vi "Main.vi"(11 "Module Admin":refnum<class "Delacor_lib_QMH_Module Admin.lvclass">) -> ()   [LabVIEW 2020, in "User Interface.lvlib"]
doc: "This template is based off of the Queued Message Handler design pattern and the Queued Message Handler project template that ships with LabVIEW.\n\nThe main difference is that the queue is private to this module and communication between modules is performed via Broadcast and Request events.\n\nRequest events are wrapped in public API methods and are handled in the Event Handling Loop (EHL) of this VI. Any module can register for Broadcast events sent by this module. The EHL generates messages based on user interface actions.\n\nThe Message Handling Loop (MHL) processes messages generated by the EHL, or by other messages. The messages are string values, so new messages can be added easily to the Message Cases case structure in the MHL. Each message cluster can also provide an optional value for Message Data, which is a variant that can be converted to whatever message-specific data is required.\n_____\nBased on Delacor QMH Project Template 6.0.0.89."
uses:
  User Interface.lvlib
  <vilib>/Delacor/Delacor QMH/Libraries/Module Admin_class/Delacor_lib_QMH_Module Admin.lvclass
  Module Data--cluster.ctl
  Stop Argument--cluster.ctl
  <vilib>/Delacor/Delacor QMH/Libraries/Message Queue_class/Delacor_lib_QMH_Message Queue.lvclass/Delacor_lib_QMH_Message Queue.ctl
  <vilib>/Delacor/Delacor QMH/Libraries/Module Admin_class/Delacor_lib_QMH_Module Admin.lvclass/Delacor_lib_QMH_Module Admin.ctl
  Start Acquisition Argument--cluster.ctl
  Settings Argument--cluster.ctl
  <vilib>/Delacor/Delacor QMH/Libraries/Message Queue_class/Delacor_lib_QMH_Enqueue Message (Single).vi
  <vilib>/Delacor/Delacor QMH/Libraries/Module Admin_class/Delacor_lib_QMH_Get External Launch.vi
  <vilib>/Utility/error.llb/Error Cluster From Error Code.vi
  <vilib>/ErrorRing/Error Ring.xnode
  <vilib>/Delacor/Delacor QMH/Libraries/Message Queue_class/Delacor_lib_QMH_Message Queue.lvclass
  Settings/Settings.lvlib
  Acquisition/Acquisition .lvlib
  Logging/Logging.lvlib
panel:
  out "Analog Signals":waveform(dbl)[](graph)
  out "Status":string
  out "Digital Signals":bool[](array[boolean])
  out "error out":errorcluster
  in  "Stop secuence":bool
  in  "Settings":bool
  in  "Start Secuence":bool
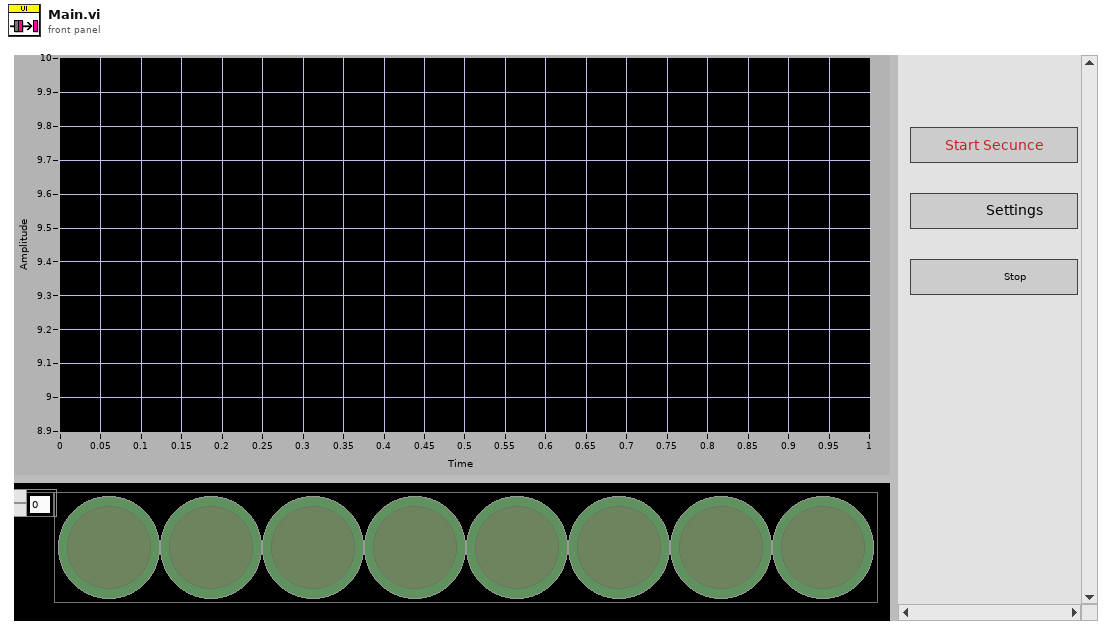
[diagram p1: front panel]
types:
  T1 = typedef "User Interface.lvlib/Request Events--cluster.ctl" = cluster{"Stop Module":refnum<user-event>, "Show Panel":refnum<user-event>, "Hide Panel":refnum<user-event>, "Get Module Execution Status":refnum<user-event>, "Show Diagram":refnum<user-event>, "Start Acquisition":refnum<user-event>, "Settings":refnum<user-event>}
  T2 = typedef "Settings.lvlib/Broadcast Events--cluster.ctl" = cluster{"Module Did Init":refnum<user-event>, "Status Updated":refnum<user-event>, "Error Reported":refnum<user-event>, "Module Did Stop":refnum<user-event>, "Update Module Execution Status":refnum<user-event>, "Config has been set":refnum<user-event>, "Prueba has been set":refnum<user-event>, "Digital has been set":refnum<user-event>}
  T3 = typedef "Acquisition .lvlib/Broadcast Events--cluster.ctl" = cluster{"Module Did Init":refnum<user-event>, "Status Updated":refnum<user-event>, "Error Reported":refnum<user-event>, "Module Did Stop":refnum<user-event>, "Update Module Execution Status":refnum<user-event>, "analog data":refnum<user-event>, "digital data":refnum<user-event>, "Digital Metdata has been acquired":refnum<user-event>}
  T4 = typedef "User Interface.lvlib/Module Data--cluster.ctl" = cluster{"Status":string}
  T5 = enum32{"invalid lock state", "Not Locked", "Locked (No Password)", "Password-protected"}
  T6 = typedef "User Interface.lvlib/Stop Argument--cluster.ctl" = cluster{"Origin":string, "Exit via Stop Module Req?":bool, "Wait for Module to stop?":bool}
  T7 = typedef "User Interface.lvlib/Start Acquisition Argument--cluster.ctl" = cluster{"Start Secuence":bool}
  T8 = typedef "User Interface.lvlib/Settings Argument--cluster.ctl" = cluster{"Settings":bool}
  T9 = enum32{"Invalid", "Standard", "Closed", "Hidden", "Minimized", "Maximized"}
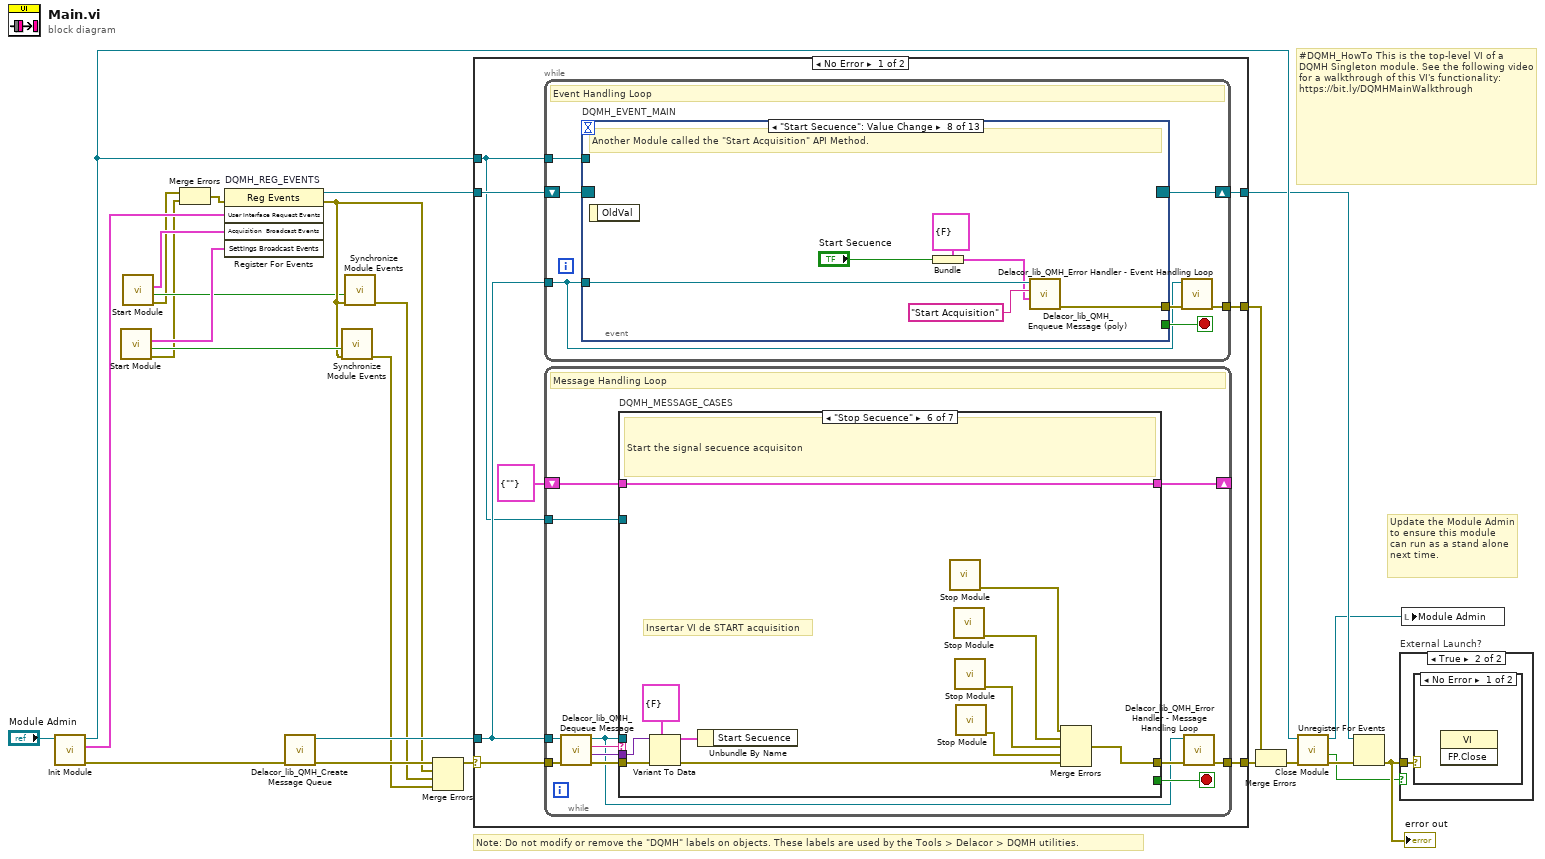
[diagram p0: block diagram]
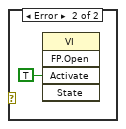
[diagram p3: hidden frame]
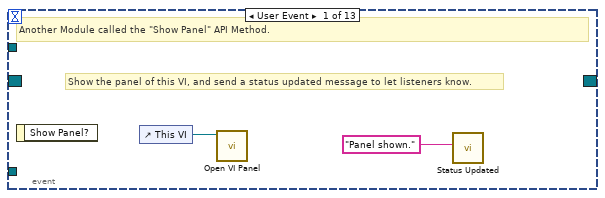
[diagram p4: hidden frame]
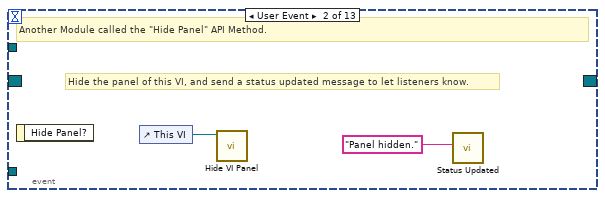
[diagram p5: hidden frame]
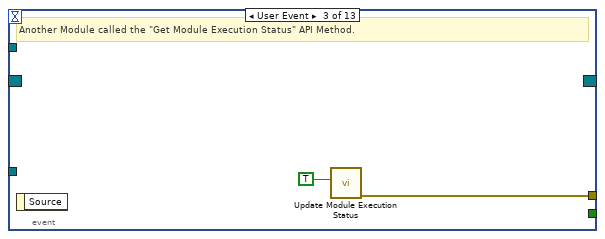
[diagram p6: hidden frame]
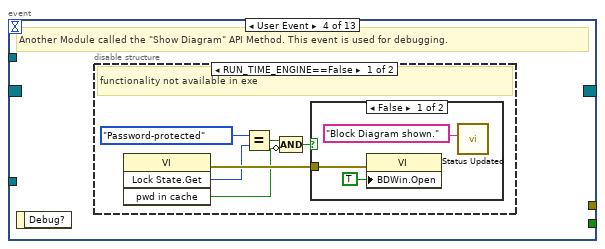
[diagram p7: hidden frame]
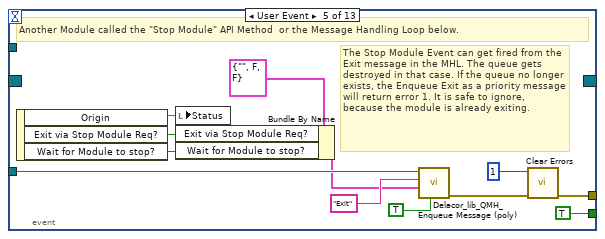
[diagram p10: hidden frame]
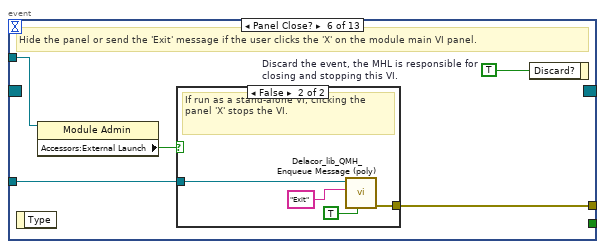
[diagram p11: hidden frame]
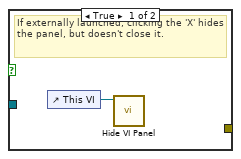
[diagram p12: hidden frame]
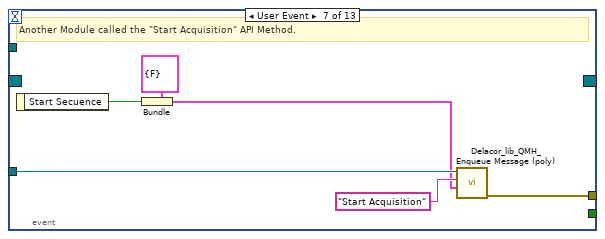
[diagram p13: hidden frame]
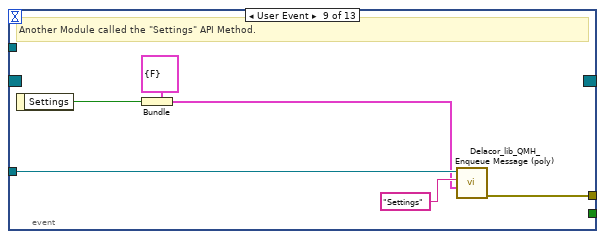
[diagram p14: hidden frame]
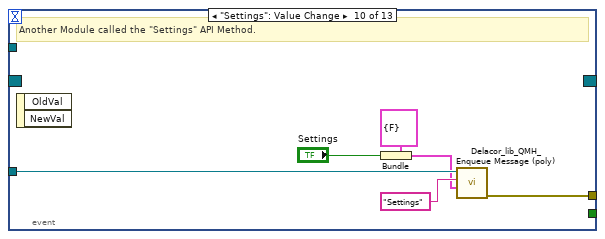
[diagram p15: hidden frame]
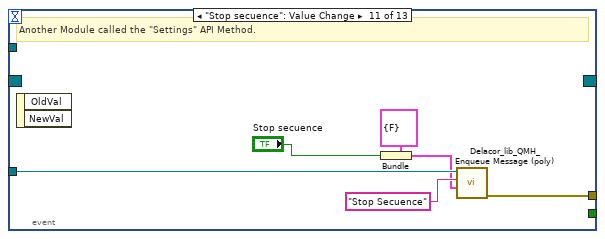
[diagram p16: hidden frame]
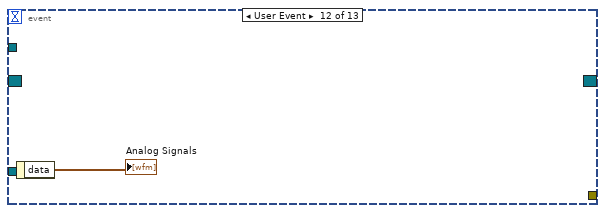
[diagram p17: hidden frame]
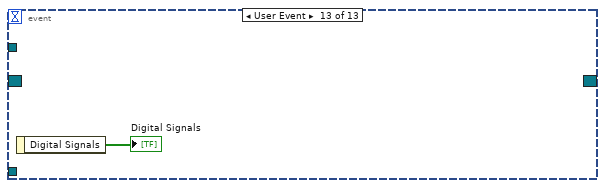
[diagram p18: hidden frame]
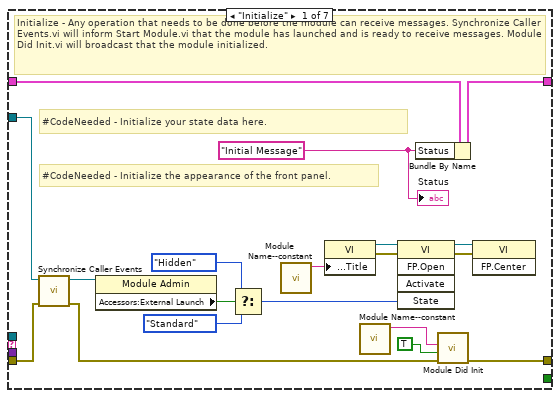
[diagram p19: hidden frame]
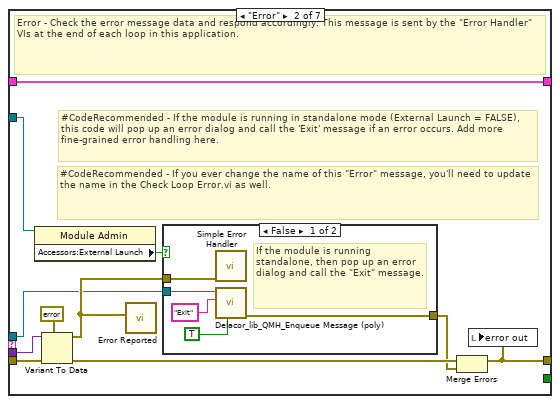
[diagram p20: hidden frame]
diagram:
  # "#DQMH_HowTo This is the top-level VI of a DQMH Singleton module. See the following video for a walkthrough of this VI's functionality: https://bit.ly/DQMHMainWalkthrough"
  # "Note: Do not modify or remove the \"DQMH\" labels on objects. These labels are used by the Tools > Delacor > DQMH utilities."
  # "Update the Module Admin to ensure this module can run as a stand alone next time."
  n1 = call "Init Module.vi"("Singleton Module Admin in"="Module Admin") -> ("error out"=w25:errorcluster, "User Interface Request Events"=w15:T1, "Singleton Module Admin out"=w18:refnum<class "Delacor_lib_QMH_Module Admin.lvclass">)  [unwired: 8 in]
  n2 = call "Start Module.vi"() -> ("error out"=w3:errorcluster, "Wait for Event Sync?"=w10:bool, "Settings Broadcast Events"=w9:T2)  [unwired: 8 in, 1 out]
  n3 = call "Start Module.vi"() -> ("error out"=w5:errorcluster, "Wait for Event Sync?"=w7:bool, "Acquisition  Broadcast Events"=w6:T3)  [unwired: 8 in, 1 out]
  n4 = Merge Errors(w5, w3) -> (w4:errorcluster)
  n5 = register-events "DQMH_REG_EVENTS"(error in=w4, w15, w6, w9) -> (reference out=w16:refnum<event-registration>, error out=w8:errorcluster)  [unwired: 1 in]
  n6 = call <vilib>:"Delacor_lib_QMH_Create Message Queue.vi"("error in"=w25) -> ("error out"=w20:errorcluster, "Message Queue"=w14:refnum<class "Delacor_lib_QMH_Message Queue.lvclass">)  [unwired: 9 in]
  n7 = call "Synchronize Module Events.vi"("error in"=w8, "Wait for Event Sync?"=w10) -> ("error out"=w2:errorcluster)  [unwired: 9 in]
  n8 = call "Synchronize Module Events.vi"("error in"=w8, "Wait for Event Sync?"=w7) -> ("error out"=w1:errorcluster)  [unwired: 9 in]
  n9 = Merge Errors(w20, w8, w1, w2) -> (w19:errorcluster)
  n10 = case shown="No Error" w19 {
    selector: w19 -> [w32 w216]
    tunnel: [w34 w215] -> w26
    tunnel: [w31 w221] -> w17
    tunnel: w16 -> [w29 w221]
    tunnel: w14 -> [w28 w214]
    tunnel: [w33 _] -> w23
    tunnel: w18 -> [w27 w217]
    frame No Error {
      n11 = while {
        tunnel: w28 -> [w35]
        shift-right: [w38] -> w31
        shift-left: w29 -> [w39]
        tunnel: [w40] -> w33
        tunnel: w27 -> [w36]
        stop <- w37 stop-if-true
        # "Event Handling Loop"
        n12 = event "DQMH_EVENT_MAIN" shown="[7] \"Start Secuence\": Value Change" {
          selector: w39 -> [_ _ _ _ _ _ _ _ _ _ _ _ _]
          dyn-events: [_ _ _ _ _ _ _ _ _ _ _ _ _] -> w38
          timeout: _ -> [_ _ _ _ _ _ _ _ _ _ _ _ _]
          tunnel: [_ _ _ _ TRUE ("Discard?") _ _ _ _ _ _ _ _] -> w37
          tunnel: w35 -> [_ _ _ _ w64 w71 w84 w90 w96 w102 w108 _ _]
          tunnel: [_ _ w47 _ w67 w73 w79 w86 w91 w98 w104 _ _] -> w41
          tunnel: w36 -> [_ _ _ _ _ w70 _ _ _ _ _ _ _]
          event User Event {
            # "Show the panel of this VI, and send a status updated message to let listeners know."
            # "Another Module called the \"Show Panel\" API Method."
            n13 = event-data() -> ()  [unwired: 1 in, 1 out]
            n14 = control-ref of="This VI"() -> (w43:refnum<vi>)
            n15 = call "Open VI Panel.vi"("VI"=w43) -> ()  [unwired: 10 in, 1 out]
            n16 = call "Status Updated.vi"("Status"="Panel shown." ("format string")) -> ()  [unwired: 10 in, 1 out]
          }
          event User Event {
            # "Hide the panel of this VI, and send a status updated message to let listeners know."
            # "Another Module called the \"Hide Panel\" API Method."
            n17 = event-data() -> ()  [unwired: 1 in, 1 out]
            n18 = control-ref of="This VI"() -> (w45:refnum<vi>)
            n19 = call "Hide VI Panel.vi"("VI"=w45) -> ()  [unwired: 10 in, 1 out]
            n20 = call "Status Updated.vi"("Status"="Panel hidden." ("format string")) -> ()  [unwired: 10 in, 1 out]
          }
          event User Event {
            # "Another Module called the \"Get Module Execution Status\" API Method."
            n21 = event-data() -> ()  [unwired: 1 in, 1 out]
            n22 = call "Update Module Execution Status.vi"("Running?"=TRUE) -> ("error out"=w47:errorcluster)  [unwired: 10 in]
          }
          event User Event {
            # "Another Module called the \"Show Diagram\" API Method. This event is used for debugging."
            n23 = event-data() -> ()  [unwired: 1 in, 1 out]
            n24 = disable-structure shown="RUN_TIME_ENGINE==False" {
              frame condition #0 (active) {
                # "functionality not available in exe"
                n25 = invoke class="VI" method="Lock State.Get"() -> (error out=w53:errorcluster, "Get Lock State"=w52:T5, "pwd in cache"=w49:bool)  [unwired: 4 in, 1 out]
                n26 = Equal?(x=T5."Password-protected", y=w52) -> (x = y?=w50:bool)
                n27 = Compound Arithmetic op=AND(w50, invert w49) -> (w48:bool)
                n28 = case shown="False" w48 {
                  tunnel: w53 -> [w56 _]
                  frame False {
                    n29 = property class="VI"(error in=w56, "BDWin.Open"=TRUE ("Block Diagram Window:Open")) -> ()  [unwired: 1 in, 2 out]
                    n30 = call "Status Updated.vi"("Status"="Block Diagram shown." ("format string")) -> ()  [unwired: 10 in, 1 out]
                  }
                  frame True {
                    # "Password-protected VI, and the password is not in the cache. Do not show the diagram."
                  }
                }
              }
              frame condition #1 {
              }
            }
          }
          event User Event {
            # "The Stop Module Event can get fired from the Exit message in the MHL. The queue gets destroyed in that case. If the queue no longer exists, the Enqueue Exit as a priority message will return error 1. It is safe to ignore, because the module is already exiting."
            # "Another Module called the \"Stop Module\" API Method  or the Message Handling Loop below."
            n31 = event-data() -> ("Origin"=w63:string, "Exit via Stop Module Req?"=w59:bool, "Wait for Module to stop?"=w58:bool)  [unwired: 1 in]
            n32 = local write "Status"(w63) -> ()
            n33 = Bundle By Name(cluster=T6 {"Origin"="", "Exit via Stop Module Req?"=FALSE, "Wait for Module to stop?"=FALSE} ("Stop Argument"), "Exit via Stop Module Req?"=w59, "Wait for Module to stop?"=w58) -> (w57:T6)
            n34 = call-poly <vilib>:"Delacor_lib_QMH_Enqueue Message (poly).vi"("Priority Message? (F)"=TRUE, "Message Data"=w57, "Message"="Exit", "Message Queue in"=w64) -> ("error out"=w68:errorcluster)  [unwired: 6 in, 1 out]
            n35 = call <vilib>:"Clear Errors.vi"("error in (no error)"=w68, "specific error code to clear (0: all)"=1) -> ("error out"=w67:errorcluster)  [unwired: 4 in, 1 out]
          }
          event Panel Close? {
            w72 = TRUE  # Discard the event, the MHL is responsible for closing and stopping this VI.
            # "Hide the panel or send the 'Exit' message if the user clicks the 'X' on the module main VI panel."
            n36 = event-data() -> ()  [unwired: 1 in, 1 out]
            n37 = property class="Module Admin"(reference=w70) -> ("Accessors:External Launch"=w69:bool)  [unwired: 1 in, 2 out]
            n38 = case shown="False" w69 {
              tunnel: w71 -> [_ w77]
              tunnel: [_ w78] -> w73
              frame True {
                # "If externally launched, clicking the 'X' hides the panel, but doesn't close it."
                n39 = control-ref of="This VI"() -> (w74:refnum<vi>)
                n40 = call "Hide VI Panel.vi"("VI"=w74) -> ()  [unwired: 10 in, 1 out]
              }
              frame False {
                # "If run as a stand-alone VI, clicking the panel 'X' stops the VI."
                n41 = call-poly <vilib>:"Delacor_lib_QMH_Enqueue Message (poly).vi"("Priority Message? (F)"=TRUE, "Message"="Exit", "Message Queue in"=w77) -> ("error out"=w78:errorcluster)  [unwired: 7 in, 1 out]
              }
            }
            n42 = event-data("Discard?"=w72) -> ()  [unwired: 1 in, 1 out]
          }
          event User Event {
            # "Another Module called the \"Start Acquisition\" API Method."
            n43 = event-data() -> ("Start Secuence"=w80:bool)  [unwired: 1 in]
            n44 = Bundle(cluster=T7 {"Start Secuence"=FALSE} ("Start Acquisition Argument"), "Start Secuence"=w80) -> (w81:T7)
            n45 = call-poly <vilib>:"Delacor_lib_QMH_Enqueue Message (poly).vi"("Message Data"=w81, "Message"="Start Acquisition", "Message Queue in"=w84) -> ("error out"=w79:errorcluster)  [unwired: 7 in, 1 out]
          }
          event "Start Secuence": Value Change {
            # "Another Module called the \"Start Acquisition\" API Method."
            n46 = event-data() -> ()  [unwired: 1 in, 1 out]
            n47 = Bundle(cluster=T7 {"Start Secuence"=FALSE} ("Start Acquisition Argument"), "Start Secuence"="Start Secuence") -> (w87:T7)
            n48 = call-poly <vilib>:"Delacor_lib_QMH_Enqueue Message (poly).vi"("Message Data"=w87, "Message"="Start Acquisition", "Message Queue in"=w90) -> ("error out"=w86:errorcluster)  [unwired: 7 in, 1 out]
          }
          event User Event {
            # "Another Module called the \"Settings\" API Method."
            n49 = event-data() -> ("Settings"=w92:bool)  [unwired: 1 in]
            n50 = Bundle(cluster=T8 {"Settings"=FALSE} ("Settings Argument"), "Settings"=w92) -> (w93:T8)
            n51 = call-poly <vilib>:"Delacor_lib_QMH_Enqueue Message (poly).vi"("Message Data"=w93, "Message"="Settings", "Message Queue in"=w96) -> ("error out"=w91:errorcluster)  [unwired: 7 in, 1 out]
          }
          event "Settings": Value Change {
            # "Another Module called the \"Settings\" API Method."
            n52 = event-data() -> ()  [unwired: 1 in, 2 out]
            n53 = Bundle(cluster=T8 {"Settings"=FALSE} ("Settings Argument"), "Settings"="Settings") -> (w99:T8)
            n54 = call-poly <vilib>:"Delacor_lib_QMH_Enqueue Message (poly).vi"("Message Data"=w99, "Message"="Settings", "Message Queue in"=w102) -> ("error out"=w98:errorcluster)  [unwired: 7 in, 1 out]
          }
          event "Stop secuence": Value Change {
            # "Another Module called the \"Settings\" API Method."
            n55 = event-data() -> ()  [unwired: 1 in, 2 out]
            n56 = Bundle(cluster=T8 {"Settings"=FALSE} ("Settings Argument"), "Settings"="Stop secuence") -> (w105:T8)
            n57 = call-poly <vilib>:"Delacor_lib_QMH_Enqueue Message (poly).vi"("Message Data"=w105, "Message"="Stop Secuence", "Message Queue in"=w108) -> ("error out"=w104:errorcluster)  [unwired: 7 in, 1 out]
          }
          event User Event {
            n58 = event-data() -> ("data"=→"Analog Signals":waveform(dbl)[])  [unwired: 1 in]
          }
          event User Event {
            n59 = event-data() -> ("Digital Signals"=→"Digital Signals":bool[])  [unwired: 1 in]
          }
        }
        n60 = call-dynamic "Delacor_lib_QMH_Error Handler - Event Handling Loop.vi"("error in"=w41, "Message Queue in"=w35) -> ("dup error in"=w40:errorcluster)  [unwired: 8 in, 1 out]
      }
      n61 = while {
        tunnel: w28 -> [w113]
        shift-right: [w117] -> _
        shift-left: T4 {"Status"=""} ("Data Cluster") -> [w118]
        tunnel: w32 -> [w121]
        tunnel: [w119] -> w34
        tunnel: w27 -> [w111]
        stop <- w116 stop-if-true
        # "Message Handling Loop"
        n62 = call-dynamic "Delacor_lib_QMH_Dequeue Message.vi"("error in"=w121, "Message Queue in"=w113) -> ("error out"=w120:errorcluster, "Message Data"=w114:variant, "Message"=w115:string, "Message Queue out"=w112:refnum<class "Delacor_lib_QMH_Message Queue.lvclass">)  [unwired: 6 in]
        n63 = case "DQMH_MESSAGE_CASES" shown="\"Stop Secuence\"" w115 {
          selector: w115 -> [_ _ _ w174 _ _ _]
          tunnel: w112 -> [_ w144 w166 _ _ _ _]
          tunnel: w120 -> [w139 w151 w172 w176 w194 w205 w213]
          tunnel: [w137 w147 w169 w177 w188 w199 w207] -> w122
          tunnel: w118 -> [w128 w146 w165 w175 w193 w204 w212]
          tunnel: [w127 w146 w165 w175 w193 w204 w212] -> w117
          tunnel: [_ _ w164 _ _ _ _] -> w116
          tunnel: w114 -> [_ w145 w163 _ w191 w202 w210]
          tunnel: w111 -> [w129 w143 w158 _ _ _ _]
          frame "Initialize" {
            w123 = "Initial Message" ("Initial Message")
            # "#CodeNeeded - Initialize the appearance of the front panel."
            # "#CodeNeeded - Initialize your state data here."
            # "Initialize - Any operation that needs to be done before the module can receive messages. Synchronize Caller Events.vi will inform Start Module.vi that the module has launched and is ready to receive messages. Module Did Init.vi will broadcast that the module initialized."
            n64 = call "Synchronize Caller Events.vi"("error in (no error)"=w139, "Singleton Module Admin in"=w129) -> ("error out"=w138:errorcluster, "Singleton Module Admin out"=w124:refnum<class "Delacor_lib_QMH_Module Admin.lvclass">)  [unwired: 8 in]
            n65 = property class="Module Admin"(reference=w124) -> ("Accessors:External Launch"=w133:bool)  [unwired: 1 in, 2 out]
            n66 = Select(t=T9."Hidden" ("State"), s=w133, f=T9."Standard" ("State")) -> (s? t:f=w130:T9)
            n67 = call "Module Name--constant.vi"() -> ("Module Name"=w136:string)  [unwired: 11 in]
            n68 = property class="VI"("Front Panel.Title"=w136) -> (reference out=w135:refnum<vi>, error out=w141:errorcluster)  [unwired: 2 in]
            n69 = call "Module Name--constant.vi"() -> ("Module Name"=w125:string)  [unwired: 11 in]
            n70 = invoke class="VI" method="FP.Open"(reference=w135, error in=w141, "State"=w130) -> (reference out=w134:refnum<vi>, error out=w140:errorcluster)  [unwired: 2 in, 3 out]
            n71 = Bundle By Name(cluster=w128, "Status"=w123) -> (w127:T4)
            n72 = call "Module Did Init.vi"("error in (no error)"=w138, "Initialized?"=TRUE, "Origin"=w125) -> ("error out"=w137:errorcluster)  [unwired: 8 in]
            n73 = invoke class="VI" method="FP.Center"(reference=w134, error in=w140) -> ()  [unwired: 1 in, 3 out]
            "Status" <- w123
          }
          frame "Error" {
            # "#CodeRecommended - If you ever change the name of this \"Error\" message, you'll need to update the name in the Check Loop Error.vi as well."
            # "#CodeRecommended - If the module is running in standalone mode (External Launch = FALSE), this code will pop up an error dialog and call the 'Exit' message if an error occurs. Add more fine-grained error handling here."
            # "Error - Check the error message data and respond accordingly. This message is sent by the \"Error Handler\" VIs at the end of each loop in this application."
            n74 = property class="Module Admin"(reference=w143) -> ("Accessors:External Launch"=w142:bool)  [unwired: 1 in, 2 out]
            n75 = Variant To Data(error in=w151, type=errorcluster {"status"=FALSE, "code"=0, "source"=""} ("error constant"), Variant=w145) -> (data=w152:errorcluster, error out=w149:errorcluster)
            n76 = call "Error Reported.vi"("Error"=w152) -> ()  [unwired: 10 in, 1 out]
            n77 = case shown="False" w142 {
              tunnel: [w157 _] -> w148
              tunnel: w144 -> [w155 _]
              tunnel: w152 -> [w156 _]
              frame False {
                # "If the module is running standalone, then pop up an error dialog and call the \"Exit\" message."
                n78 = call <vilib>:"Simple Error Handler.vi"("error in (no error)"=w156) -> ()  [unwired: 4 in, 5 out]
                n79 = call-poly <vilib>:"Delacor_lib_QMH_Enqueue Message (poly).vi"("Priority Message? (F)"=TRUE, "Message"="Exit", "Message Queue in"=w155) -> ("error out"=w157:errorcluster)  [unwired: 7 in, 1 out]
              }
              frame True {
                # "If the module was launched externally, calling the Error Reported broadcast VI is the only action performed by the \"Error\" message. The module's caller can then process the error appropriately."
              }
            }
            n80 = Merge Errors(w149, w148) -> (w147:errorcluster)
            n81 = local write "error out"(w147) -> ()
          }
          frame "Exit" {
            w162 = 91  # 91: not all Exit messages will have an argument
            w164 = TRUE  # Stop the VI
            # "Release the message queue reference"
            # "#CodeNeeded - Add any required cleanup code here"
            # "Exit - Exit the application."
            n82 = Variant To Data(error in=w172, type=T6 {"Origin"="", "Exit via Stop Module Req?"=FALSE, "Wait for Module to stop?"=FALSE} ("Stop Argument"), Variant=w163) -> (data=w160:T6, error out=w168:errorcluster)
            n83 = call <vilib>:"Clear Errors.vi"("error in (no error)"=w168, "specific error code to clear (0: all)"=w162) -> ("error out"=w171:errorcluster)  [unwired: 4 in, 1 out]
            n84 = control-ref of="This VI"() -> (w159:refnum<vi>)
            n85 = call-dynamic "Delacor_lib_QMH_Release Message Queue.vi"("error in"=w171, "Message Queue"=w166) -> ("error out"=w170:errorcluster)  [unwired: 9 in]
            n86 = call "Handle Exit.vi"("Stop Argument"=w160, "Admin in"=w158, "VI reference"=w159) -> ("error out"=w167:errorcluster)  [unwired: 7 in, 1 out]
            n87 = Merge Errors(w170, w167) -> (w169:errorcluster)
          }
          frame Default {
            # "'Default' case only runs if there is a message that isn't defined in any of the other cases.  Output a programming error."
            n88 = call "Module Name--constant.vi"() -> ("Module Name"=w173:string)  [unwired: 11 in]
            n89 = xnode "Error Ring"("parameter 0"=w174, "parameter 1"=w173) -> ("error out"=w178:errorcluster)
            n90 = Merge Errors(w176, w178) -> (w177:errorcluster)
          }
          frame "Start Acquisition" {
            # "Insertar VI de START acquisition"
            # "Start the signal secuence acquisiton"
            n91 = Variant To Data(error in=w194, type=T7 {"Start Secuence"=FALSE} ("Start Acquisition Argument"), Variant=w191) -> (data=w189:T7, error out=w192:errorcluster)
            n92 = Unbundle By Name(w189) -> ()  [unwired: 1 out]
            n93 = call "Start Helper Loop.vi"() -> ("error out"=w187:errorcluster)  [unwired: 11 in]
            n94 = Merge Errors(w187, w192) -> (w188:errorcluster)
          }
          frame "Stop Secuence" {
            # "Insertar VI de START acquisition"
            # "Start the signal secuence acquisiton"
            n95 = Variant To Data(error in=w205, type=T7 {"Start Secuence"=FALSE} ("Start Acquisition Argument"), Variant=w202) -> (data=w200:T7, error out=w203:errorcluster)
            n96 = Unbundle By Name(w200) -> ()  [unwired: 1 out]
            n97 = call "Stop Module.vi"() -> ("error out"=w195:errorcluster)  [unwired: 11 in]
            n98 = call "Stop Module.vi"() -> ("error out"=w196:errorcluster)  [unwired: 11 in]
            n99 = call "Stop Module.vi"() -> ("error out"=w197:errorcluster)  [unwired: 11 in]
            n100 = call "Stop Module.vi"() -> ("error out"=w198:errorcluster)  [unwired: 11 in]
            n101 = Merge Errors(w195, w196, w197, w198, w203) -> (w199:errorcluster)
          }
          frame "Settings" {
            # "Insertar VI de setting SHOW Panel"
            # "Open the Settings VI"
            n102 = Variant To Data(error in=w213, type=T8 {"Settings"=FALSE} ("Settings Argument"), Variant=w210) -> (data=w208:T8, error out=w211:errorcluster)
            n103 = Unbundle By Name(w208) -> ()  [unwired: 1 out]
            n104 = call "Show Panel.vi"() -> ("error out"=w206:errorcluster)  [unwired: 11 in]
            n105 = Merge Errors(w206, w211) -> (w207:errorcluster)
          }
        }
        n106 = call-dynamic "Delacor_lib_QMH_Error Handler - Message Handling Loop.vi"("error in"=w122, "Message Queue in"=w112) -> ("dup error in"=w119:errorcluster)  [unwired: 8 in, 1 out]
      }
    }
    frame Error {
      # "Synchronize Caller Events.vi will inform Start Module.vi that the module has launched and will let the code calling Start Module.vi register for broadcasts and would permit the caller receive the broadcast that an error occurred at launch time."
      n107 = call-dynamic "Delacor_lib_QMH_Release Message Queue.vi"("error in"=w216, "Message Queue"=w214) -> ("error out"=w215:errorcluster)  [unwired: 9 in]
      n108 = call "Synchronize Caller Events.vi"("Singleton Module Admin in"=w217) -> ("error out"=w222:errorcluster)  [unwired: 9 in, 1 out]
      n109 = call "Module Name--constant.vi"() -> ("Module Name"=w220:string)  [unwired: 11 in]
      n110 = Format Into String(format string="An error occurred during initialization. %s is no longer running.", w220) -> (resulting string=w218:string)  [unwired: 2 in, 1 out]
      n111 = Merge Errors(w215, w222) -> (w223:errorcluster)
      n112 = call "Error Reported.vi"("Additional Information"=w218, "Error"=w223) -> ()  [unwired: 9 in, 1 out]
      n113 = call "Stop Module.vi"() -> ()  [unwired: 11 in, 1 out]
      n114 = call "Stop Module.vi"() -> ()  [unwired: 11 in, 1 out]
    }
  }
  n115 = Merge Errors(w23, w26) -> (w22:errorcluster)
  n116 = call "Close Module.vi"("error in (no error)"=w22, "Module Admin in"=w18) -> ("error out"=w24:errorcluster, "External Launch"=w11:bool, "Module Admin out"=w12:refnum<class "Delacor_lib_QMH_Module Admin.lvclass">)  [unwired: 7 in]
  n117 = Unregister For Events(event registration refnum=w17, error in=w24) -> (error out=w21:errorcluster)
  "error out" <- w21
  n118 = case "External Launch?" shown="True" w11 {
    tunnel: w21 -> [_ w224]
    frame False {
    }
    frame True {
      n119 = case shown="No Error" w224 {
        frame No Error {
          n120 = invoke class="VI" method="FP.Close"() -> ()  [unwired: 3 in, 3 out]
        }
        frame Error {
          n121 = invoke class="VI" method="FP.Open"("Activate"=TRUE ("Activate?")) -> ()  [unwired: 4 in, 5 out]
        }
      }
    }
  }
  n122 = local write "Module Admin"(w12) -> ()
